vi "reward_behavior_michelle_visjitter_conswinAdapt_enticefx.vi"() -> ()   [LabVIEW 2019]
doc: "The myRIO Project template acquires acceleration data from the onboard accelerometer and displays the changes of acceleration values in a waveform chart."
uses:
  <vilib>/Analysis/Matrix/Datatypes/RealMatrix.ctl
  <vilib>/myRIO/Common/Instrument Driver Framework/myRIO v1.0/Encoder/typedefs/Encoder Signal Mode.ctl
  <vilib>/myRIO/Instrument Drivers/Onboard IO/Encoder/typedefs/Encoder Reference.ctl
  <vilib>/myRIO/Common/Instrument Driver Framework/Utilities/typedefs/myRIO Generic Hardware Reference.ctl
  <vilib>/myRIO/Common/Instrument Driver Framework/Utilities/typedefs/Hardware Version Enum.ctl
  <vilib>/myRIO/Common/Instrument Driver Framework/Utilities/typedefs/myRIO v1.0 Reference.ctl
  <vilib>/myRIO/Common/Instrument Driver Framework/Utilities/typedefs/Generic FPGA Reference.ctl
  <vilib>/myRIO/Common/Instrument Driver Framework/myRIO v1.0/Encoder/typedefs/Encoder Channels Enum.ctl
  <vilib>/myRIO/Common/Instrument Driver Framework/myRIO v1.0/Encoder/typedefs/Encoder Configuration v1.0.ctl
  <vilib>/userdefined/High Color/nirio_resource_hc.ctl
  <vilib>/myRIO/Instrument Drivers/Onboard IO/DIO/typedefs/DIO Reference.ctl
  <vilib>/myRIO/Common/Instrument Driver Framework/myRIO v1.0/DIO/typedefs/DIO Channels List.ctl
  <vilib>/myRIO/Common/Instrument Driver Framework/myRIO v1.0/DIO/typedefs/DIO Channels Enum.ctl
  <vilib>/myRIO/Common/Instrument Driver Framework/Utilities/vis/Is FPGA Ref Available.vi
  <vilib>/myRIO/Common/Instrument Driver Framework/myRIO v1.0/Encoder/vis/myRIO v1.1 Open Encoder.vi
  <vilib>/myRIO/Instrument Drivers/Onboard IO/Encoder/vis/Read.vi
  <vilib>/myRIO/Common/Instrument Driver Framework/myRIO v1.0/DIO/vis/myRIO v1.1 Open DIO.vi
  <vilib>/myRIO/Instrument Drivers/Onboard IO/DIO/vis/Write.vi
  <vilib>/myRIO/Instrument Drivers/Onboard IO/DIO/vis/Read.vi
  <vilib>/myRIO/Common/Instrument Driver Framework/Utilities/vis/Validate Channels.vi
  <vilib>/myRIO/Common/Instrument Driver Framework/myRIO v1.0/Encoder/vis/myRIO v1.0 Reserve Encoder.vi
  <vilib>/myRIO/Common/Instrument Driver Framework/myRIO v1.0/DIO/vis/myRIO v1.0 Reserve DIO.vi
  <vilib>/myRIO/Common/Instrument Driver Framework/myRIO v1.0/Encoder/vis/myRIO v1.0 Build MUX Configuration Encoder.vi
  <vilib>/myRIO/Common/Instrument Driver Framework/myRIO v1.0/Resource Manager/vis/myRIO v1.0 Reserve Channel List.vi
  <vilib>/myRIO/Common/Instrument Driver Framework/myRIO v1.0/DIO/vis/myRIO v1.0 Build MUX Configuration DIO.vi
  <vilib>/myRIO/Common/Instrument Driver Framework/myRIO v1.0/Resource Manager/vis/myRIO v1.0 Create Configuration List.vi
  <vilib>/myRIO/Common/Instrument Driver Framework/myRIO v1.0/Resource Manager/vis/myRIO v1.0 Reserve Channel.vi
  <vilib>/myRIO/Common/Instrument Driver Framework/myRIO v1.0/Resource Manager/vis/myRIO v1.0 Unreserve Channel.vi
  <vilib>/myRIO/Common/Instrument Driver Framework/myRIO v1.0/Resource Manager/vis/myRIO v1.0 Build Mutex Name.vi
  <vilib>/Utility/VariantDataType/GetNumericInfo.vi
  <vilib>/Utility/error.llb/Error Cluster From Error Code.vi
  <vilib>/myRIO/Common/Instrument Driver Framework/myRIO v1.0/myRIO v1.1 Open.vi
  <vilib>/myRIO/Common/Instrument Driver Framework/Utilities/vis/IO Manager.vi
  <vilib>/myRIO/Common/Instrument Driver Framework/Utilities/vis/Configuration Manager.vi
  <vilib>/myRIO/Common/Instrument Driver Framework/myRIO v1.0/Resource Manager/vis/myRIO v1.0 Configure IO.vi
  <vilib>/myRIO/Common/Instrument Driver Framework/myRIO v1.0/myRIO v1.0 Close.vi
  <vilib>/myRIO/Common/Instrument Driver Framework/myRIO v1.0/Encoder/vis/myRIO v1.0 Configure Encoder.vi
  <vilib>/myRIO/Common/Instrument Driver Framework/myRIO v1.0/Encoder/vis/myRIO v1.0 Read Encoder.vi
  GlobalVars.vi
  <vilib>/myRIO/Common/Instrument Driver Framework/myRIO v1.0/DIO/vis/myRIO v1.0 Read DIO.vi
  <vilib>/myRIO/Common/Instrument Driver Framework/myRIO v1.0/DIO/vis/myRIO v1.0 Write DIO.vi
  <vilib>/myRIO/Express VI/Onboard IO/Encoder/Encoder Express VI.xnode
  <vilib>/myRIO/Instrument Drivers/Onboard IO/Encoder/vis/myRIO Encoder Open.xnode
  <vilib>/myRIO/Express VI/Onboard IO/DI/DI Express VI.xnode
  <vilib>/myRIO/Instrument Drivers/Onboard IO/DIO/vis/myRIO DIO Open.xnode
  <vilib>/myRIO/Express VI/Onboard IO/DO/DO Express VI.xnode
  <vilib>/myRIO/Instrument Drivers/Onboard IO/Encoder/Encoder.lvlib
  <vilib>/myRIO/Instrument Drivers/Onboard IO/DIO/DIO.lvlib
  <vilib>/Analysis/Matrix/NI_Matrix.lvlib
panel:
  out "LAG":dbl
  out "ContrastChoice":dbl
  out "Its":i32
  out "BurstCriteria":dbl
  out "LickBurst 2":bool
  out "LickBurst":bool
  out "Enticements":i32
  in  "Entice":bool
  out "Misses":i32
  out "GoAhead":bool
  out "TimeOutDuration":i32
  out "ActiveTime":dbl
  out "ConsumptionGo":bool=TRUE
  out "Consumption_Period":i32
  out "Watch_Display":bool=TRUE
  in  "Give reward":bool
  out "Timings":dbl[](array[numeric])
  out "ISI":dbl
  out "ISI start time":dbl
  out "Time_out":bool=TRUE
  out "Time since lick":dbl
  out "Time of last lick":dbl
  out "Rewarded trials":dbl[](array[numeric])
  out "Rewards":u16
  out "Active Trial":bool
  out "Array temp2":T1
  out "Stimuli Loaded":bool
  out "Stim_ID":dbl[](array[numeric])
  out "Reward_mat":dbl[](array[numeric])
  out "Reward":bool=TRUE
  out "Frame clock":i32
  out "Licks":u32
  out "Lick":bool
  out "Time":dbl
  out "Stop":bool
  in  "Frames to collect":u32
  out "Overflow?":bool
  out "Counter Value":i32
  out "Velocity":dbl
  out "Velocity Plot":dbl[](graph)
  out "Velocity array":dbl[](array[numeric])
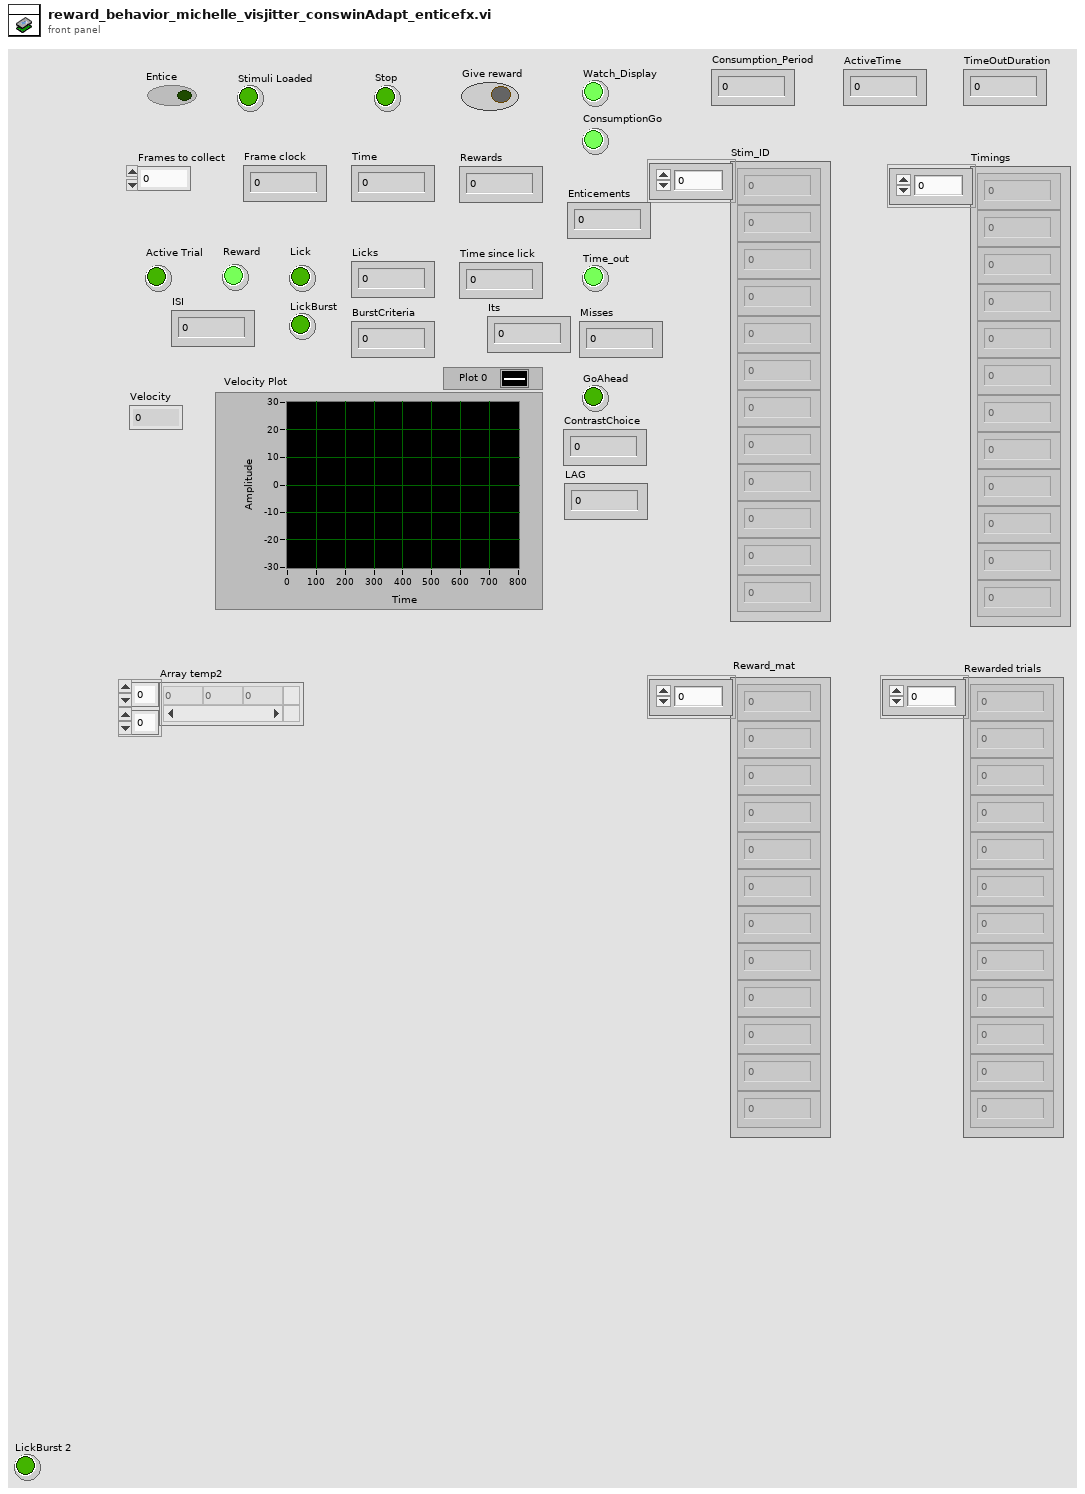
[diagram p1: front panel]
types:
  T1 = typedef "NI_Matrix.lvlib/RealMatrix.ctl" = dbl[][]
  T2 = typedef "Encoder.lvlib/Encoder Reference.ctl" = cluster{"myRIO Reference":T3, "Encoder Channels Enum":T7}
  T3 = typedef "myRIO Generic Hardware Reference.ctl" = cluster{"myRIO Model":T4, "myRIO Hardware Reference":T5}
  T4 = typedef "Hardware Version Enum.ctl" = enum16{"Unknown", "myRIO-1900", "myRIO-1950", "roboRIO", "NI ELVIS RIO CM", "ELVIS III"}
  T5 = typedef "myRIO v1.0 Reference.ctl" = cluster{"Generic FPGA Reference":T6, "Allow multiple opens":bool}
  T6 = typedef "Generic FPGA Reference.ctl" = refnum<k20>
  T7 = typedef "Encoder Channels Enum.ctl" = enum16{"Not Connected", "C/ENC0", "C/ENC1", "A/ENC", "A/ENC0", "A/ENC1", "A/ENC2", "A/ENC3", "A/ENC4", "A/ENC5", "A/ENC6", "A/ENC7", "A/ENC8", "A/ENC9", "B/ENC", "B/ENC0", "B/ENC1", "B/ENC2", "B/ENC3", "B/ENC4", "B/ENC5", "B/ENC6", "B/ENC7", "B/ENC8", "B/ENC9", "DIO/ENC0", "DIO/ENC1", "DIO/ENC2", "DIO/ENC3", "DIO/ENC4"}
  T8 = typedef "Encoder Signal Mode.ctl" = enum16{"Quadrature phase signal", "Step and direction signal"}
  T9 = typedef "nirio_resource_hc.ctl" = tag
  T10 = typedef "DIO.lvlib/DIO Reference.ctl" = cluster{"myRIO Reference":T3, "DIO Channels List":T11}
  T11 = typedef "DIO Channels List.ctl" = T12[]
  T12 = typedef "DIO Channels Enum.ctl" = enum16{"Not Connected", "C/DIO0", "C/DIO1", "C/DIO2", "C/DIO3", "C/DIO4", "C/DIO5", "C/DIO6", "C/DIO7", "A/DIO0", "A/DIO1", "A/DIO2", "A/DIO3", "A/DIO4", "A/DIO5", "A/DIO6", "A/DIO7", "A/DIO8", "A/DIO9", "A/DIO10", "A/DIO11", "A/DIO12", "A/DIO13", "A/DIO14", "A/DIO15", "A/DIO16", "A/DIO17", "A/DIO18", "A/DIO19", "B/DIO0", "B/DIO1", "B/DIO2", "B/DIO3", "B/DIO4", "B/DIO5", "B/DIO6", "B/DIO7", "B/DIO8", "B/DIO9", "B/DIO10", "B/DIO11", "B/DIO12", "B/DIO13", "B/DIO14", "B/DIO15", "B/DIO16", "B/DIO17", "B/DIO18", "B/DIO19", "LED0", "LED1", "LED2", "LED3", "Button0", "DIO/DIO0", "DIO/DIO1", "DIO/DIO2", "DIO/DIO3", "DIO/DIO4", "DIO/DIO5", "DIO/DIO6", "DIO/DIO7", "DIO/DIO8", "DIO/DIO9", "SPI/CS0", "SPI/CS1", "SPI/CS2", "SPI/CS3", "LED RADIO (Green)", "LED RADIO (Red)", "LED COMM (Green)", "LED COMM (Red)", "LED MODE (Green)", "LED MODE (Red)"}
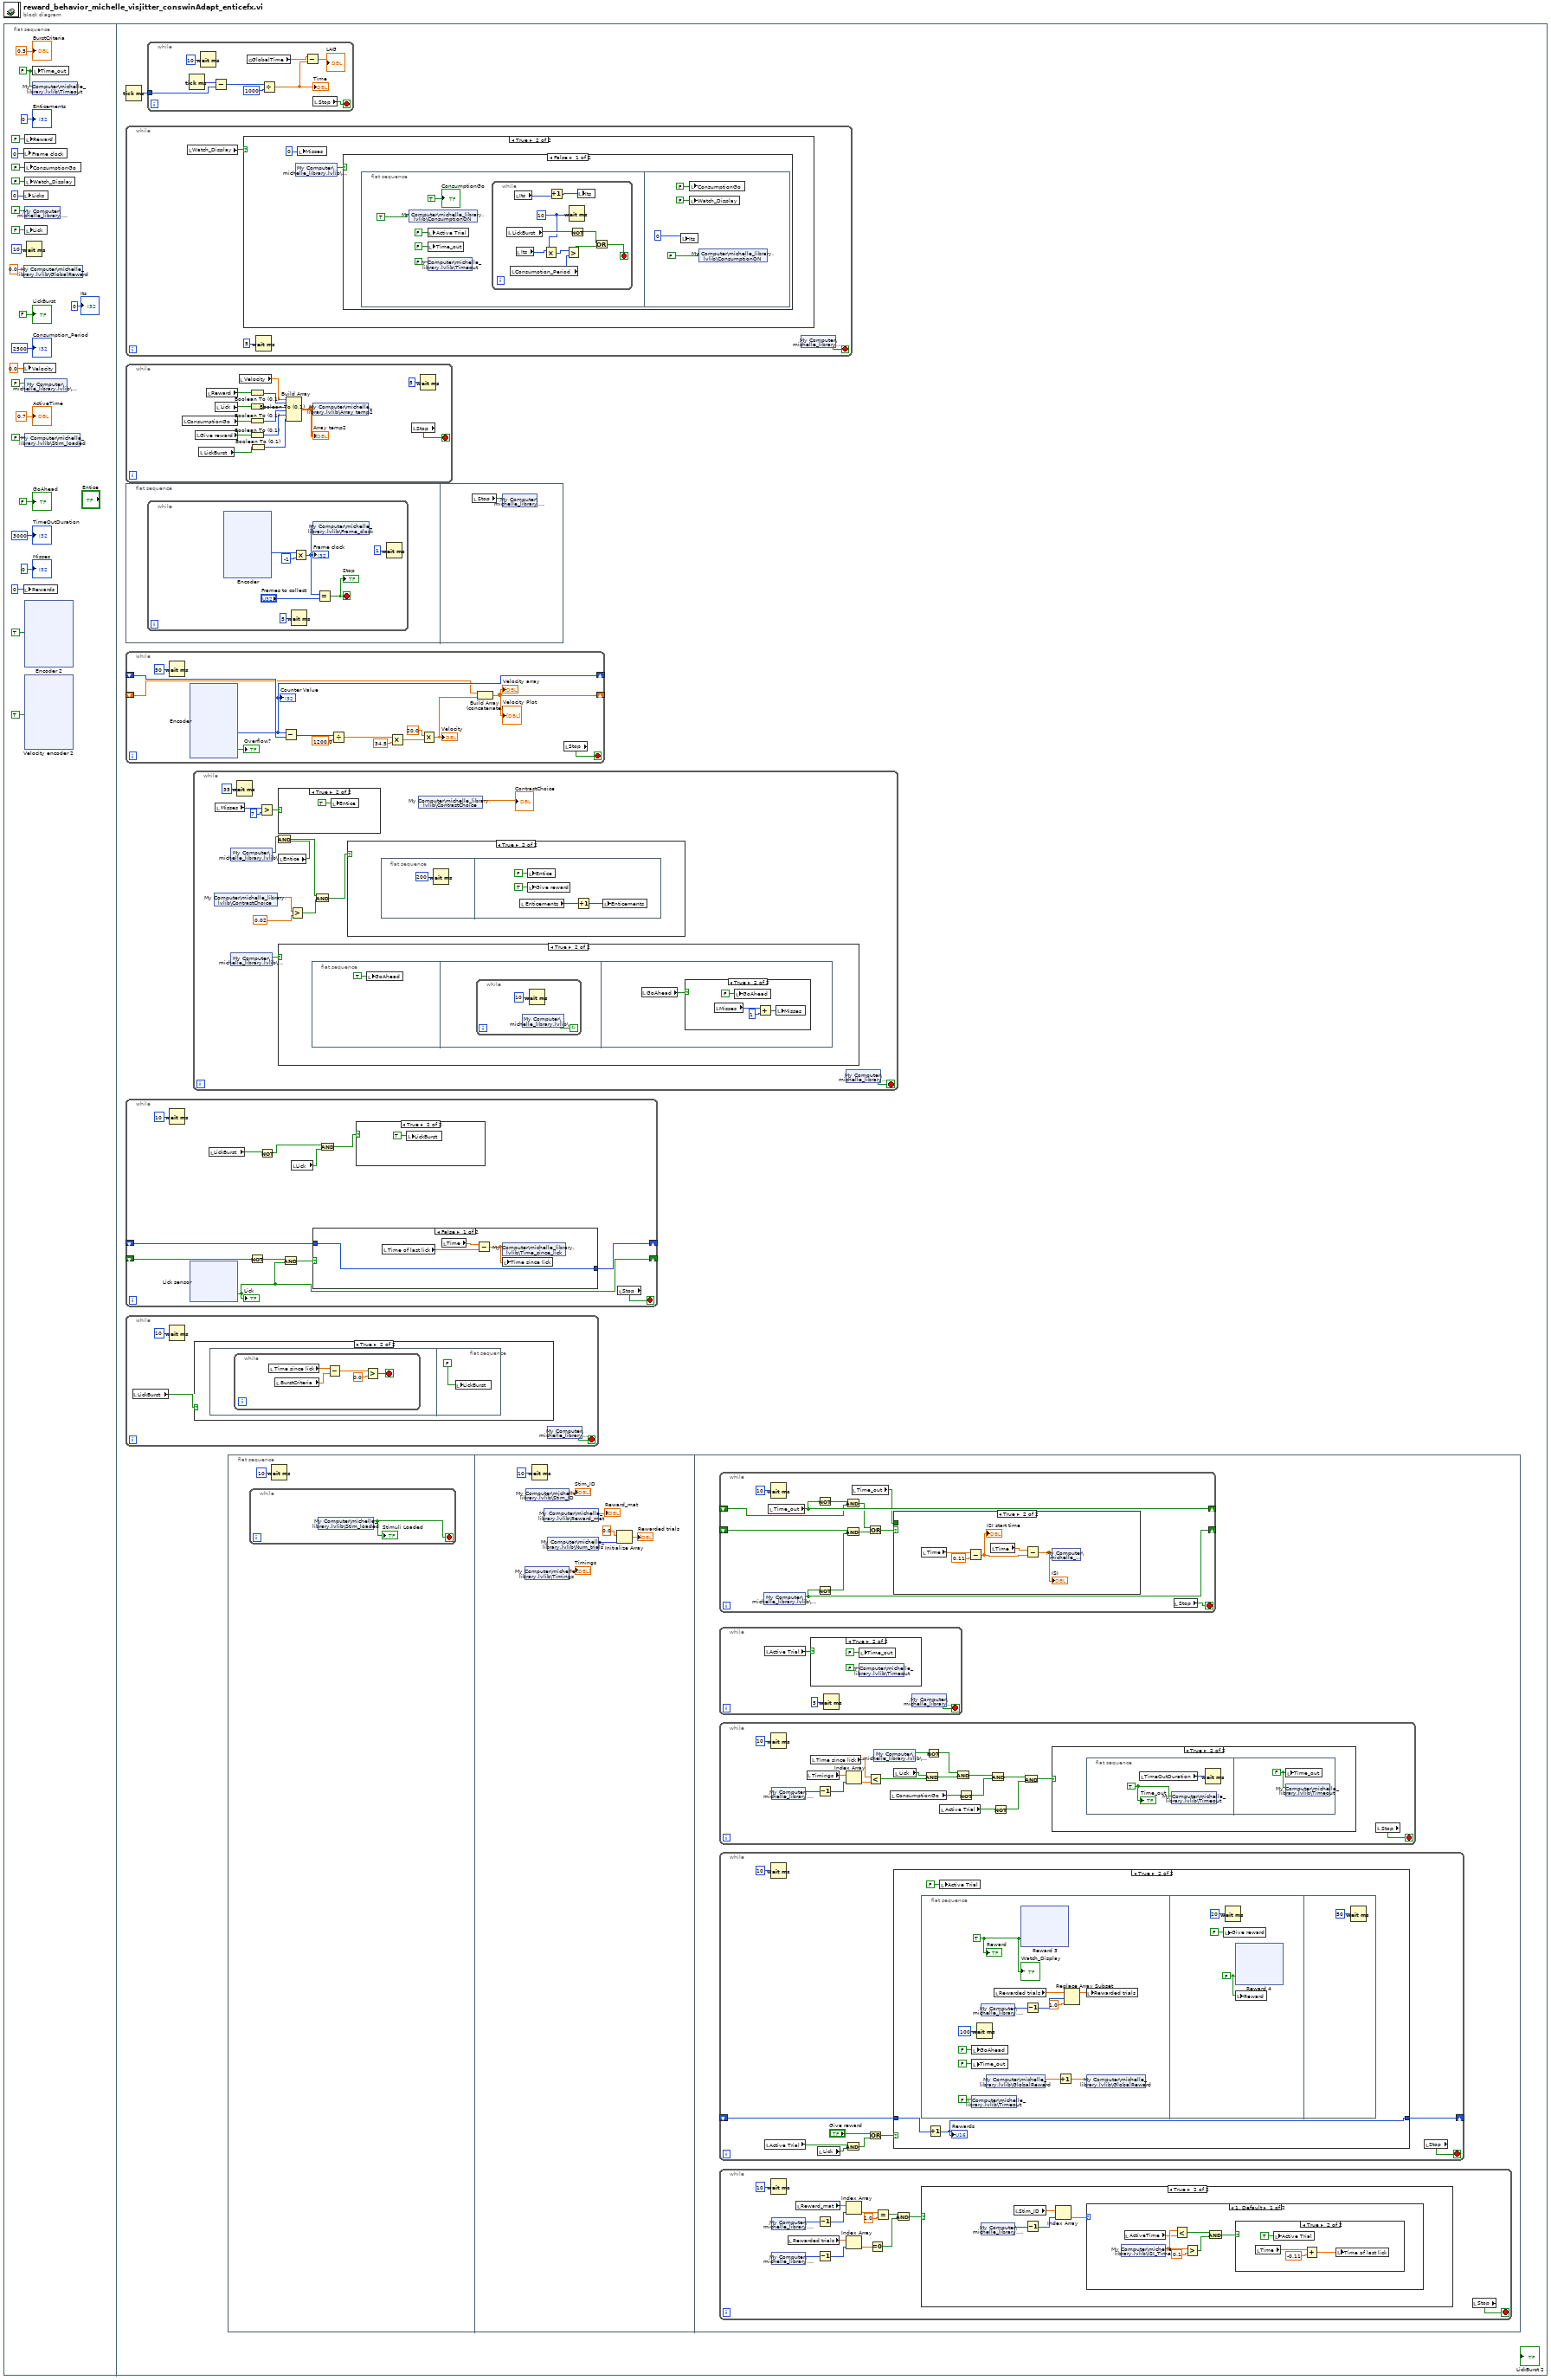
[diagram p0: block diagram]
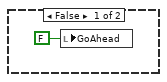
[diagram p5: hidden frame]
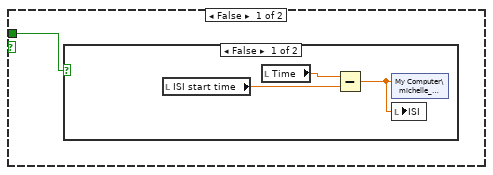
[diagram p11: hidden frame]
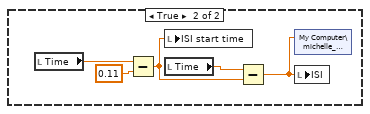
[diagram p12: hidden frame]
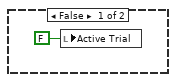
[diagram p13: hidden frame]
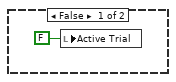
[diagram p14: hidden frame]
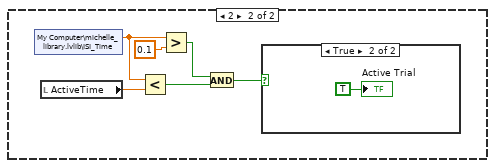
[diagram p15: hidden frame]
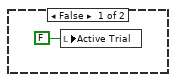
[diagram p16: hidden frame]
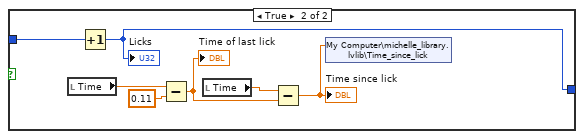
[diagram p19: hidden frame]
diagram:
  n1 = flat-sequence {
    frame #0 {
      w13 = FALSE ("Time_out")
      n2 = local write "Frame clock"(u32 0 ("Frames")) -> ()
      n3 = local write "Licks"(u32 0 ("Licks")) -> ()
      n4 = shared-variable "My Computer\\michelle_library.lvlib\\GlobalReward"(0.0) -> ()  [unwired: 1 in, 1 out]
      n5 = local write "Velocity"(0.0 ("Velocity")) -> ()
      n6 = local write "Rewards"(u16 0 ("Rewards")) -> ()
      n7 = local write "Reward"(FALSE ("Give reward")) -> ()
      n8 = local write "ConsumptionGo"(FALSE ("ConsumptionGo")) -> ()
      n9 = local write "Watch_Display"(FALSE ("Watch_Display")) -> ()
      n10 = shared-variable "My Computer\\michelle_library.lvlib\\Stop"(FALSE ("Stop")) -> ()  [unwired: 1 in, 1 out]
      n11 = local write "Lick"(FALSE ("Lick")) -> ()
      n12 = shared-variable "My Computer\\michelle_library.lvlib\\Display"(FALSE ("Display")) -> ()  [unwired: 1 in, 1 out]
      n13 = shared-variable "My Computer\\michelle_library.lvlib\\Stim_loaded"(FALSE ("Stim_loaded")) -> ()  [unwired: 1 in, 1 out]
      n14 = xnode "Encoder 2"("Reset Counter"=TRUE) -> ()  [unwired: 1 in, 4 out]
      n15 = xnode "Velocity encoder 2"("Reset Counter"=TRUE) -> ()  [unwired: 1 in, 4 out]
      n16 = Wait (ms)(milliseconds to wait=u32 10) -> ()  [unwired: 1 out]
      n17 = local write "Time_out"(w13) -> ()
      n18 = shared-variable "My Computer\\michelle_library.lvlib\\Timeout"(w13) -> ()  [unwired: 1 in, 1 out]
      "Consumption_Period" <- 2500
      "ActiveTime" <- 0.7
      "TimeOutDuration" <- 3000
      "GoAhead" <- FALSE
      "Misses" <- 0
      "Enticements" <- 0
      "LickBurst" <- FALSE
      "BurstCriteria" <- 0.5
      "Its" <- 0
    }
    frame #1 {
      n19 = Tick Count (ms)() -> (millisecond timer value=w118:u32)
      n20 = while {
        stop <- w159 stop-if-true
        n21 = local read "Watch_Display"() -> (w158:bool)
        n22 = case shown="True" w158 {
          frame False {
          }
          frame True {
            n23 = shared-variable "My Computer\\michelle_library.lvlib\\Display"() -> (w161:bool)  [unwired: 1 in, 1 out]
            n24 = local write "Misses"(0) -> ()
            n25 = case shown="False" w161 {
              frame False {
                n26 = flat-sequence {
                  frame #0 {
                    n27 = shared-variable "My Computer\\michelle_library.lvlib\\ConsumptionON"(TRUE) -> ()  [unwired: 1 in, 1 out]
                    n28 = local write "Active Trial"(FALSE) -> ()
                    n29 = local write "Time_out"(FALSE) -> ()
                    n30 = shared-variable "My Computer\\michelle_library.lvlib\\Timeout"(FALSE) -> ()  [unwired: 1 in, 1 out]
                    n31 = while {
                      stop <- w170 stop-if-true
                      w171 = 10
                      n32 = local read "LickBurst"() -> (w176:bool)
                      n33 = local read "Consumption_Period"() -> (w168:i32)
                      n34 = local read "Its"() -> (w175:i32)
                      n35 = local read "Its"() -> (w172:i32)
                      n36 = Multiply(x=w172, y=w171) -> (x*y=w169:i32)
                      n37 = Increment(x=w175) -> (x+1=w174:i32)
                      n38 = Greater?(x=w169, y=w168) -> (0:w167:bool)
                      n39 = Wait (ms)(milliseconds to wait=w171) -> ()  [unwired: 1 out]
                      n40 = Not(x=w176) -> (.not. x?=w173:bool)
                      n41 = local write "Its"(w174) -> ()
                      n42 = Or(x=w173, y=w167) -> (x .or. y?=w170:bool)
                    }
                    "ConsumptionGo" <- TRUE
                  }
                  frame #1 {
                    n43 = local write "Its"(0) -> ()
                    n44 = local write "ConsumptionGo"(FALSE ("ConsumptionGo")) -> ()
                    n45 = local write "Watch_Display"(FALSE ("Watch_Display")) -> ()
                    n46 = shared-variable "My Computer\\michelle_library.lvlib\\ConsumptionON"(FALSE) -> ()  [unwired: 1 in, 1 out]
                  }
                }
              }
              frame True {
              }
            }
          }
        }
        n47 = Wait (ms)(milliseconds to wait=u32 5) -> ()  [unwired: 1 out]
        n48 = shared-variable "My Computer\\michelle_library.lvlib\\Stop"() -> (w159:bool)  [unwired: 1 in, 1 out]
      }
      n49 = while {
        stop <- w188 stop-if-true
        n50 = local read "ConsumptionGo"() -> (w186:bool)
        n51 = local read "Give reward"() -> (w185:bool)
        n52 = local read "LickBurst"() -> (w182:bool)
        n53 = local read "Reward"() -> (w193:bool)
        n54 = local read "Lick"() -> (w194:bool)
        n55 = local read "Velocity"() -> (w192:dbl)
        n56 = Boolean To (0,1)(Boolean=w193) -> (0, 1=w191:i16)
        n57 = Boolean To (0,1)(Boolean=w194) -> (0, 1=w190:i16)
        n58 = Boolean To (0,1)(Boolean=w186) -> (0, 1=w184:i16)
        n59 = Boolean To (0,1)(Boolean=w185) -> (0, 1=w183:i16)
        n60 = Boolean To (0,1)(Boolean=w182) -> (0, 1=w181:i16)
        n61 = Build Array(w192, w191, w190, w184, w183, w181) -> (w187:T1)
        "Array temp2" <- w187
        n62 = shared-variable "My Computer\\michelle_library.lvlib\\Array temp2"(w187) -> ()  [unwired: 1 in, 1 out]
        n63 = local read "Stop"() -> (w188:bool)
        n64 = Wait (ms)(milliseconds to wait=u32 5) -> ()  [unwired: 1 out]
      }
      n65 = flat-sequence {
        frame #0 {
          n66 = while {
            stop <- w395 stop-if-true
            n67 = xnode "Encoder"() -> ("Counter Value"=w399:i32)  [unwired: 2 in, 3 out]
            n68 = Wait (ms)(milliseconds to wait=u32 5) -> ()  [unwired: 1 out]
            n69 = Multiply(x=w399, y=-1) -> (x*y=w394:i32)
            "Frame clock" <- w394
            n70 = shared-variable "My Computer\\michelle_library.lvlib\\Frame_clock"(w394) -> ()  [unwired: 1 in, 1 out]
            n71 = Equal?(x=w394, y="Frames to collect") -> (x = y?=w395:bool)
            "Stop" <- w395
            n72 = Wait (ms)(milliseconds to wait=u32 1) -> ()  [unwired: 1 out]
          }
        }
        frame #1 {
          n73 = local read "Stop"() -> (w447:bool)
          n74 = shared-variable "My Computer\\michelle_library.lvlib\\Stop"(w447) -> ()  [unwired: 1 in, 1 out]
        }
      }
      n75 = while {
        shift-right: [w517] -> _
        shift-left: _ -> [w518]
        shift-right: [w509] -> _
        shift-left: _ -> [w508]
        stop <- w507 stop-if-true
        n76 = Wait (ms)(milliseconds to wait=u32 50) -> ()  [unwired: 1 out]
        n77 = xnode "Encoder"() -> ("Counter Value"=w517:i32, "Overflow?"=→"Overflow?":bool)  [unwired: 2 in, 2 out]
        "Counter Value" <- w517
        n78 = Subtract(x=w517, y=w518) -> (x-y=w510:i32)
        n79 = Divide(x=w510, y=1200.0 ("600")) -> (x/y=w515:dbl)
        n80 = Multiply(x=w515, y=34.5) -> (x*y=w513:dbl)
        n81 = Multiply(x=20.0, y=w513) -> (x*y=w511:dbl)
        "Velocity" <- w511
        n82 = Build Array (concatenate)(w508, w511) -> (w509:dbl[])
        "Velocity Plot" <- w509
        "Velocity array" <- w509
        n83 = local read "Stop"() -> (w507:bool)
      }
      n84 = while {
        shift-right: [w458] -> _
        shift-left: _ -> [w457]
        shift-right: [w452] -> _
        shift-left: _ -> [w455]
        stop <- w456 stop-if-true
        n85 = Wait (ms)(milliseconds to wait=u32 10) -> ()  [unwired: 1 out]
        n86 = xnode "Lick sensor"() -> ("C/DIO1 (DIO1)"=w452:bool)  [unwired: 1 in, 1 out]
        "Lick" <- w452
        n87 = local read "LickBurst"() -> (w449:bool)
        n88 = Not(x=w455) -> (.not. x?=w454:bool)
        n89 = Not(x=w449) -> (.not. x?=w448:bool)
        n90 = And(x=w454, y=w452) -> (x .and. y?=w453:bool)
        n91 = local read "Lick"() -> (w450:bool)
        n92 = case shown="False" w453 {
          tunnel: [w464 w471] -> w458
          tunnel: w457 -> [w464 w470]
          frame False {
            n93 = local read "Time of last lick"() -> (w462:dbl)
            n94 = local read "Time"() -> (w463:dbl)
            n95 = Subtract(x=w463, y=w462) -> (x-y=w461:dbl)
            n96 = shared-variable "My Computer\\michelle_library.lvlib\\Time_since_lick"(w461) -> ()  [unwired: 1 in, 1 out]
            n97 = local write "Time since lick"(w461) -> ()
          }
          frame True {
            n98 = local read "Time"() -> (w467:dbl)
            n99 = Increment(x=w470) -> (x+1=w471:u32)
            "Licks" <- w471
            n100 = Subtract(x=w467, y=0.11) -> (x-y=w465:dbl)
            "Time of last lick" <- w465
            n101 = local read "Time"() -> (w469:dbl)
            n102 = Subtract(x=w469, y=w465) -> (x-y=w468:dbl)
            "Time since lick" <- w468
            n103 = shared-variable "My Computer\\michelle_library.lvlib\\Time_since_lick"(w468) -> ()  [unwired: 1 in, 1 out]
          }
        }
        n104 = And(x=w448, y=w450) -> (x .and. y?=w451:bool)
        n105 = case shown="True" w451 {
          frame False {
          }
          frame True {
            n106 = local write "LickBurst"(TRUE) -> ()
          }
        }
        n107 = local read "Stop"() -> (w456:bool)
      }
      n108 = while {
        stop <- w121 stop-if-true
        n109 = local read "LickBurst"() -> (w119:bool)
        n110 = Wait (ms)(milliseconds to wait=u32 10) -> ()  [unwired: 1 out]
        n111 = case shown="True" w119 {
          frame False {
          }
          frame True {
            n112 = flat-sequence {
              frame #0 {
                n113 = while {
                  stop <- w124 stop-if-true
                  n114 = local read "Time since lick"() -> (w125:dbl)
                  n115 = local read "BurstCriteria"() -> (w126:dbl)
                  n116 = Subtract(x=w125, y=w126) -> (x-y=w122:dbl)
                  n117 = Greater?(x=w122, y=0.0) -> (0:w124:bool)
                }
              }
              frame #1 {
                n118 = local write "LickBurst"(FALSE) -> ()
              }
            }
          }
        }
        n119 = shared-variable "My Computer\\michelle_library.lvlib\\Stop"() -> (w121:bool)  [unwired: 1 in, 1 out]
      }
      n120 = while {
        tunnel: w118 -> [w574]
        stop <- w572 stop-if-true
        n121 = Tick Count (ms)() -> (millisecond timer value=w575:u32)
        n122 = Wait (ms)(milliseconds to wait=u32 10) -> ()  [unwired: 1 out]
        n123 = Subtract(x=w575, y=w574) -> (x-y=w571:u32)
        n124 = global read "GlobalVars.vi" "GlobalTime"() -> (w569:dbl)
        n125 = Divide(x=w571, y=u32 1000) -> (x/y=w568:dbl)
        "Time" <- w568
        n126 = Subtract(x=w569, y=w568) -> (x-y=→"LAG":dbl)
        n127 = local read "Stop"() -> (w572:bool)
      }
      n128 = while {
        stop <- w141 stop-if-true
        n129 = shared-variable "My Computer\\michelle_library.lvlib\\ContrastChoice"() -> (w132:dbl)  [unwired: 1 in, 1 out]
        n130 = local read "Misses"() -> (w139:i32)
        n131 = shared-variable "My Computer\\michelle_library.lvlib\\Display"() -> (w136:bool)  [unwired: 1 in, 1 out]
        n132 = shared-variable "My Computer\\michelle_library.lvlib\\Display"() -> (w140:bool)  [unwired: 1 in, 1 out]
        n133 = Wait (ms)(milliseconds to wait=35) -> ()  [unwired: 1 out]
        n134 = Greater?(x=w139, y=7) -> (0:w137:bool)
        n135 = case shown="True" w137 {
          frame False {
          }
          frame True {
            n136 = local write "Entice"(TRUE) -> ()
          }
        }
        n137 = local read "Entice"() -> (w135:bool)
        n138 = And(x=w136, y=w135) -> (x .and. y?=w133:bool)
        n139 = case shown="True" w140 {
          frame False {
            n140 = local write "GoAhead"(FALSE) -> ()
          }
          frame True {
            n141 = flat-sequence {
              frame #0 {
                n142 = local write "GoAhead"(TRUE) -> ()
              }
              frame #1 {
                n143 = while {
                  stop <- w151 continue-if-true
                  n144 = shared-variable "My Computer\\michelle_library.lvlib\\Display"() -> (w151:bool)  [unwired: 1 in, 1 out]
                  n145 = Wait (ms)(milliseconds to wait=10) -> ()  [unwired: 1 out]
                }
              }
              frame #2 {
                n146 = local read "GoAhead"() -> (w152:bool)
                n147 = case shown="True" w152 {
                  frame False {
                  }
                  frame True {
                    n148 = local read "Misses"() -> (w156:i32)
                    n149 = local write "GoAhead"(FALSE) -> ()
                    n150 = Add(x=w156, y=1) -> (x+y=w154:i32)
                    n151 = local write "Misses"(w154) -> ()
                  }
                }
              }
            }
          }
        }
        n152 = Greater?(x=w132, y=0.02) -> (0:w131:bool)
        n153 = And(x=w133, y=w131) -> (x .and. y?=w130:bool)
        n154 = case shown="True" w130 {
          frame False {
          }
          frame True {
            n155 = flat-sequence {
              frame #0 {
                n156 = Wait (ms)(milliseconds to wait=200) -> ()  [unwired: 1 out]
              }
              frame #1 {
                n157 = local read "Enticements"() -> (w144:i32)
                n158 = local write "Entice"(FALSE) -> ()
                n159 = local write "Give reward"(TRUE) -> ()
                n160 = Increment(x=w144) -> (x+1=w143:i32)
                n161 = local write "Enticements"(w143) -> ()
              }
            }
          }
        }
        n162 = shared-variable "My Computer\\michelle_library.lvlib\\ContrastChoice"() -> (→"ContrastChoice":dbl)  [unwired: 1 in, 1 out]
        n163 = shared-variable "My Computer\\michelle_library.lvlib\\Stop"() -> (w141:bool)  [unwired: 1 in, 1 out]
      }
      n164 = flat-sequence {
        frame #0 {
          n165 = while {
            stop <- w196 stop-if-true
            n166 = shared-variable "My Computer\\michelle_library.lvlib\\Stim_loaded"() -> (w196:bool)  [unwired: 1 in, 1 out]
            "Stimuli Loaded" <- w196
          }
          n167 = Wait (ms)(milliseconds to wait=u32 10) -> ()  [unwired: 1 out]
        }
        frame #1 {
          n168 = shared-variable "My Computer\\michelle_library.lvlib\\Timings"() -> (→"Timings":dbl[])  [unwired: 1 in, 1 out]
          n169 = shared-variable "My Computer\\michelle_library.lvlib\\Stim_ID"() -> (→"Stim_ID":dbl[])  [unwired: 1 in, 1 out]
          n170 = Wait (ms)(milliseconds to wait=u32 10) -> ()  [unwired: 1 out]
          n171 = shared-variable "My Computer\\michelle_library.lvlib\\Reward_mat"() -> (→"Reward_mat":dbl[])  [unwired: 1 in, 1 out]
          n172 = shared-variable "My Computer\\michelle_library.lvlib\\Num_trials"() -> (w200:u32)  [unwired: 1 in, 1 out]
          n173 = Initialize Array(0.0 ("element"), w200) -> (→"Rewarded trials":dbl[])
        }
        frame #2 {
          n174 = while {
            shift-right: [w241] -> _
            shift-left: _ -> [w239]
            shift-right: [w237] -> _
            shift-left: _ -> [w236]
            stop <- w242 stop-if-true
            n175 = shared-variable "My Computer\\michelle_library.lvlib\\Display"() -> (w237:bool)  [unwired: 1 in, 1 out]
            n176 = local read "Time_out"() -> (w241:bool)
            n177 = Wait (ms)(milliseconds to wait=u32 10) -> ()  [unwired: 1 out]
            n178 = Not(x=w241) -> (.not. x?=w240:bool)
            n179 = Not(x=w237) -> (.not. x?=w235:bool)
            n180 = And(x=w240, y=w239) -> (x .and. y?=w234:bool)
            n181 = And(x=w236, y=w235) -> (x .and. y?=w233:bool)
            n182 = local read "Time_out"() -> (w238:bool)
            n183 = Or(x=w234, y=w233) -> (x .or. y?=w232:bool)
            n184 = case shown="True" w232 {
              tunnel: w238 -> [w243 _]
              frame False {
                n185 = case shown="False" w243 {
                  frame False {
                    n186 = local read "ISI start time"() -> (w246:dbl)
                    n187 = local read "Time"() -> (w245:dbl)
                    n188 = Subtract(x=w245, y=w246) -> (x-y=w244:dbl)
                    n189 = shared-variable "My Computer\\michelle_library.lvlib\\ISI"(w244) -> ()  [unwired: 1 in, 1 out]
                    n190 = local write "ISI"(w244) -> ()
                  }
                  frame True {
                    n191 = local read "Time"() -> (w251:dbl)
                    n192 = Subtract(x=w251, y=0.11) -> (x-y=w248:dbl)
                    n193 = local write "ISI start time"(w248) -> ()
                    n194 = local read "Time"() -> (w249:dbl)
                    n195 = Subtract(x=w249, y=w248) -> (x-y=w247:dbl)
                    n196 = shared-variable "My Computer\\michelle_library.lvlib\\ISI"(w247) -> ()  [unwired: 1 in, 1 out]
                    n197 = local write "ISI"(w247) -> ()
                  }
                }
              }
              frame True {
                n198 = local read "Time"() -> (w256:dbl)
                n199 = Subtract(x=w256, y=0.11) -> (x-y=w253:dbl)
                "ISI start time" <- w253
                n200 = local read "Time"() -> (w254:dbl)
                n201 = Subtract(x=w254, y=w253) -> (x-y=w252:dbl)
                "ISI" <- w252
                n202 = shared-variable "My Computer\\michelle_library.lvlib\\ISI"(w252) -> ()  [unwired: 1 in, 1 out]
              }
            }
            n203 = local read "Stop"() -> (w242:bool)
          }
          n204 = while {
            stop <- w206 stop-if-true
            n205 = local read "Active Trial"() -> (w205:bool)
            n206 = case shown="True" w205 {
              frame False {
              }
              frame True {
                n207 = local write "Time_out"(FALSE) -> ()
                n208 = shared-variable "My Computer\\michelle_library.lvlib\\Timeout"(FALSE) -> ()  [unwired: 1 in, 1 out]
              }
            }
            n209 = Wait (ms)(milliseconds to wait=5) -> ()  [unwired: 1 out]
            n210 = shared-variable "My Computer\\michelle_library.lvlib\\Stop"() -> (w206:bool)  [unwired: 1 in, 1 out]
          }
          n211 = while {
            stop <- w227 stop-if-true
            n212 = Wait (ms)(milliseconds to wait=u32 10) -> ()  [unwired: 1 out]
            n213 = shared-variable "My Computer\\michelle_library.lvlib\\Trial"() -> (w217:u32)  [unwired: 1 in, 1 out]
            n214 = local read "Timings"() -> (w219:dbl[])
            n215 = local read "Time since lick"() -> (w226:dbl)
            n216 = Decrement(x=w217) -> (x-1=w216:u32)
            n217 = Index Array(array=w219, index=w216) -> (element=w218:dbl)
            n218 = Less?(x=w226, y=w218) -> (x < y?=w225:bool)
            n219 = shared-variable "My Computer\\michelle_library.lvlib\\Display"() -> (w222:bool)  [unwired: 1 in, 1 out]
            n220 = local read "ConsumptionGo"() -> (w214:bool)
            n221 = local read "Lick"() -> (w224:bool)
            n222 = And(x=w224, y=w225) -> (x .and. y?=w220:bool)
            n223 = Not(x=w222) -> (.not. x?=w221:bool)
            n224 = local read "Active Trial"() -> (w209:bool)
            n225 = And(x=w221, y=w220) -> (x .and. y?=w213:bool)
            n226 = Not(x=w214) -> (.not. x?=w215:bool)
            n227 = And(x=w213, y=w215) -> (x .and. y?=w211:bool)
            n228 = Not(x=w209) -> (.not. x?=w212:bool)
            n229 = And(x=w211, y=w212) -> (x .and. y?=w210:bool)
            n230 = case shown="True" w210 {
              frame False {
              }
              frame True {
                n231 = flat-sequence {
                  frame #0 {
                    w229 = TRUE
                    n232 = local read "TimeOutDuration"() -> (w228:i32)
                    n233 = shared-variable "My Computer\\michelle_library.lvlib\\Timeout"(w229) -> ()  [unwired: 1 in, 1 out]
                    n234 = Wait (ms)(milliseconds to wait=w228) -> ()  [unwired: 1 out]
                    "Time_out" <- w229
                  }
                  frame #1 {
                    w230 = FALSE ("Timeout")
                    n235 = local write "Time_out"(w230) -> ()
                    n236 = shared-variable "My Computer\\michelle_library.lvlib\\Timeout"(w230) -> ()  [unwired: 1 in, 1 out]
                  }
                }
              }
            }
            n237 = local read "Stop"() -> (w227:bool)
          }
          n238 = while {
            shift-right: [w301] -> _
            shift-left: _ -> [w300]
            stop <- w303 stop-if-true
            n239 = local read "Active Trial"() -> (w298:bool)
            n240 = Wait (ms)(milliseconds to wait=u32 10) -> ()  [unwired: 1 out]
            n241 = local read "Lick"() -> (w299:bool)
            n242 = And(x=w298, y=w299) -> (x .and. y?=w297:bool)
            n243 = Or(x="Give reward", y=w297) -> (x .or. y?=w296:bool)
            n244 = case shown="True" w296 {
              tunnel: [w304 w307] -> w301
              tunnel: w300 -> [w304 w306]
              frame False {
              }
              frame True {
                n245 = flat-sequence {
                  frame #0 {
                    w318 = TRUE ("C/DIO0 (DIO0)")
                    n246 = local write "GoAhead"(FALSE) -> ()
                    n247 = local write "Time_out"(FALSE) -> ()
                    n248 = shared-variable "My Computer\\michelle_library.lvlib\\Timeout"(FALSE) -> ()  [unwired: 1 in, 1 out]
                    n249 = Wait (ms)(milliseconds to wait=u32 100) -> ()  [unwired: 1 out]
                    n250 = shared-variable "My Computer\\michelle_library.lvlib\\Trial"() -> (w317:u32)  [unwired: 1 in, 1 out]
                    n251 = shared-variable "My Computer\\michelle_library.lvlib\\GlobalReward"() -> (w309:dbl)  [unwired: 1 in, 1 out]
                    n252 = local read "Rewarded trials"() -> (w315:dbl[])
                    n253 = xnode "Reward 3"("C/DIO0 (DIO0)"=w318) -> ()  [unwired: 1 in, 1 out]
                    n254 = Decrement(x=w317) -> (x-1=w316:u32)
                    n255 = Increment(x=w309) -> (x+1=w308:dbl)
                    n256 = Replace Array Subset(array=w315, new element=1.0 ("new element/subarray"), index=w316) -> (w313:dbl[])
                    n257 = local write "Rewarded trials"(w313) -> ()
                    n258 = shared-variable "My Computer\\michelle_library.lvlib\\GlobalReward"(w308) -> ()  [unwired: 1 in, 1 out]
                    "Reward" <- w318
                    "Watch_Display" <- w318
                  }
                  frame #1 {
                    w357 = FALSE ("C/DIO0 (DIO0)")
                    n259 = local write "Give reward"(FALSE ("Give reward")) -> ()
                    n260 = Wait (ms)(milliseconds to wait=u32 20) -> ()  [unwired: 1 out]
                    n261 = xnode "Reward 4"("C/DIO0 (DIO0)"=w357) -> ()  [unwired: 1 in, 1 out]
                    n262 = local write "Reward"(w357) -> ()
                  }
                  frame #2 {
                    n263 = Wait (ms)(milliseconds to wait=u32 50) -> ()  [unwired: 1 out]
                  }
                }
                n264 = Increment(x=w306) -> (x+1=w307:u16)
                "Rewards" <- w307
                n265 = local write "Active Trial"(FALSE ("Active Trial")) -> ()
              }
            }
            n266 = local read "Stop"() -> (w303:bool)
          }
          n267 = while {
            stop <- w270 stop-if-true
            n268 = Wait (ms)(milliseconds to wait=u32 10) -> ()  [unwired: 1 out]
            n269 = shared-variable "My Computer\\michelle_library.lvlib\\Trial"() -> (w266:u32)  [unwired: 1 in, 1 out]
            n270 = shared-variable "My Computer\\michelle_library.lvlib\\Trial"() -> (w262:u32)  [unwired: 1 in, 1 out]
            n271 = local read "Rewarded trials"() -> (w263:dbl[])
            n272 = local read "Reward_mat"() -> (w265:dbl[])
            n273 = Decrement(x=w266) -> (x-1=w267:u32)
            n274 = Decrement(x=w262) -> (x-1=w261:u32)
            n275 = Index Array(array=w265, index=w267) -> (element=w268:dbl)
            n276 = Index Array(array=w263, index=w261) -> (element=w260:dbl)
            n277 = Equal To 0?(x=w260) -> (x = 0?=w259:bool)
            n278 = Equal?(x=w268, y=1.0) -> (x = y?=w258:bool)
            n279 = And(x=w258, y=w259) -> (x .and. y?=w257:bool)
            n280 = case shown="True" w257 {
              frame False {
                n281 = local write "Active Trial"(FALSE ("Active_trial")) -> ()
              }
              frame True {
                n282 = shared-variable "My Computer\\michelle_library.lvlib\\Trial"() -> (w273:u32)  [unwired: 1 in, 1 out]
                n283 = local read "Stim_ID"() -> (w275:dbl[])
                n284 = Decrement(x=w273) -> (x-1=w274:u32)
                n285 = Index Array(array=w275, index=w274) -> (element=w272:dbl)
                n286 = case shown="1, Default" w272 {
                  frame 1, Default {
                    n287 = shared-variable "My Computer\\michelle_library.lvlib\\ISI_Time"() -> (w281:dbl)  [unwired: 1 in, 1 out]
                    n288 = local read "ActiveTime"() -> (w276:dbl)
                    n289 = Less?(x=w281, y=w276) -> (x < y?=w279:bool)
                    n290 = Greater?(x=w281, y=0.1) -> (0:w278:bool)
                    n291 = And(x=w279, y=w278) -> (x .and. y?=w277:bool)
                    n292 = case shown="True" w277 {
                      frame False {
                        n293 = local write "Active Trial"(FALSE ("Active Trial")) -> ()
                      }
                      frame True {
                        n294 = local read "Time"() -> (w285:dbl)
                        n295 = local write "Active Trial"(TRUE ("Active Trial")) -> ()
                        n296 = Add(x=w285, y=-0.11) -> (x+y=w283:dbl)
                        n297 = local write "Time of last lick"(w283) -> ()
                      }
                    }
                  }
                  frame 2 {
                    n298 = shared-variable "My Computer\\michelle_library.lvlib\\ISI_Time"() -> (w291:dbl)  [unwired: 1 in, 1 out]
                    n299 = local read "ActiveTime"() -> (w287:dbl)
                    n300 = Less?(x=w291, y=w287) -> (x < y?=w289:bool)
                    n301 = Greater?(x=w291, y=0.1) -> (0:w290:bool)
                    n302 = And(x=w290, y=w289) -> (x .and. y?=w288:bool)
                    n303 = case shown="True" w288 {
                      frame False {
                        n304 = local write "Active Trial"(FALSE ("Active Trial")) -> ()
                      }
                      frame True {
                        "Active Trial" <- TRUE ("Active Trial")
                      }
                    }
                  }
                }
              }
            }
            n305 = local read "Stop"() -> (w270:bool)
          }
        }
      }
    }
  }
